vi "Active By Pressing.vi"(1 "Global Data Name 1":bool, 2 "Button Press":bool) -> (0 "Global Data Name 2":bool)   [LabVIEW 2018]
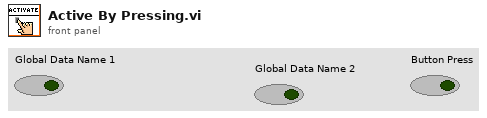
[diagram p1: front panel]
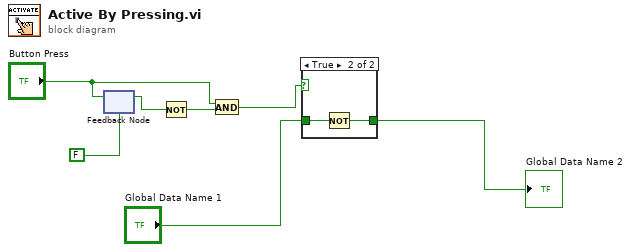
[diagram p0: block diagram]
diagram:
  n1 = feedback-in #1("Button Press") -> ()
  n2 = feedback #1(FALSE) -> (w2:bool)
  n3 = Not(x=w2) -> (.not. x?=w5:bool)
  n4 = And(x="Button Press", y=w5) -> (x .and. y?=w4:bool)
  n5 = case shown="True" w4 {
    tunnel: "Global Data Name 1" -> [w8 w10]
    tunnel: [w8 w9] -> w7
    frame False {
    }
    frame True {
      n6 = Not(x=w10) -> (.not. x?=w9:bool)
    }
  }
  "Global Data Name 2" <- w7
